vi "MeasAction.vi"(8 "error in (no error)":errorcluster caption="entrée d'erreur (pas d'erreur)", 9 "CurvePointIndex":i32, 10 "AllPointIndex":i32, 11 "DefaultDevIn":refnum<class "PhotoLum.lvclass"> caption="DNL_LabVIEW Object in") -> (0 "error out":errorcluster caption="sortie d'erreur", 2 "MeasDatOut":dbl[](array[numeric]), 3 "DefaultDevOut":refnum<class "PhotoLum.lvclass"> caption="DNL_LabVIEW Object out")   [LabVIEW 2019, in "PhotoLum.lvclass"]
uses:
  PhotoLum.lvclass
  PhotoLum.lvclass/PhotoLum.ctl
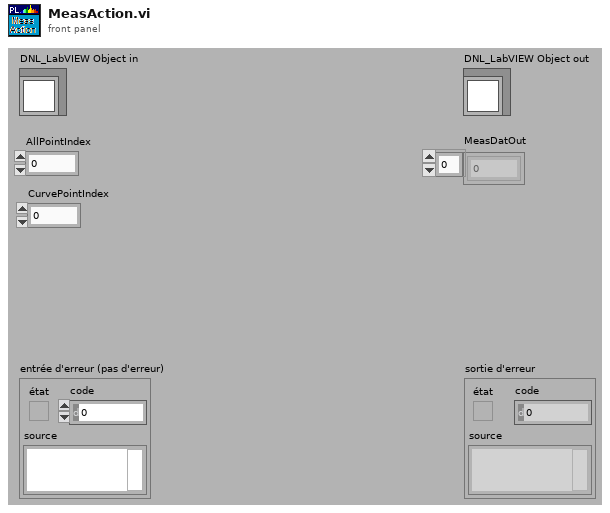
[diagram p1: front panel]
types:
  T1 = typedef "PhotoLum.lvclass/PhotoLum_Func.ctl" = enum16{"ScanInfoPanel (Na)", "MicroPLInfoPanel (NA)", "ExcimerInfoPan (NA)"}
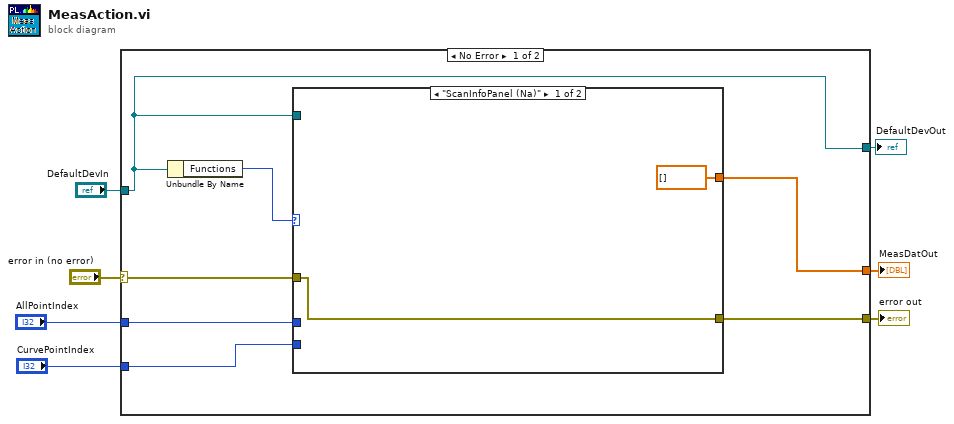
[diagram p0: block diagram]
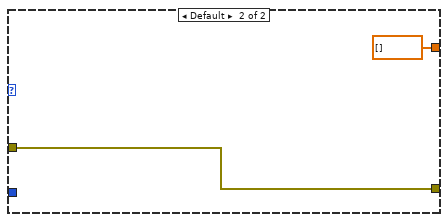
[diagram p2: hidden frame]
diagram:
  n1 = case shown="No Error" "error in (no error)" {
    selector: "error in (no error)" -> [w10 w19]
    tunnel: "DefaultDevIn" -> [w8 w20]
    tunnel: [w8 w20] -> w5
    tunnel: "AllPointIndex" -> [w14 _]
    tunnel: [w13 w19] -> w3
    tunnel: [w12 _] -> w2
    tunnel: "CurvePointIndex" -> [w9 _]
    frame No Error {
      n2 = Unbundle By Name(w8) -> ("Functions"=w11:T1)
      n3 = case shown="\"ScanInfoPanel (Na)\"" w11 {
        tunnel: w14 -> [_ _]
        tunnel: [w16 w17] -> w13
        tunnel: [dbl[] [] ("Outputs") dbl[] [] ("Outputs")] -> w12
        tunnel: w10 -> [w16 w17]
        tunnel: w9 -> [_ _]
        tunnel: w8 -> [_ _]
        frame "ScanInfoPanel (Na)" {
        }
        frame Default {
        }
      }
    }
    frame Error {
    }
  }
  "error out" <- w3
  "DefaultDevOut" <- w5
  "MeasDatOut" <- w2
